vi "XVC_TX.vi"(6 "data in":string="shift:\u0005\u0000\u0000\u0000ÿ\u0000", 7 "Read (TRUE)":bool, 8 "error in":errorcluster, 9 "Address":u32=64 format="%.0x", 10 "IP address":string="192.168.10.20", 11 "connection ID":refnum<k16>) -> (0 "error out":errorcluster, 2 "received string":string, 3 "connection ID 2":refnum<k16>)   [LabVIEW 2017]
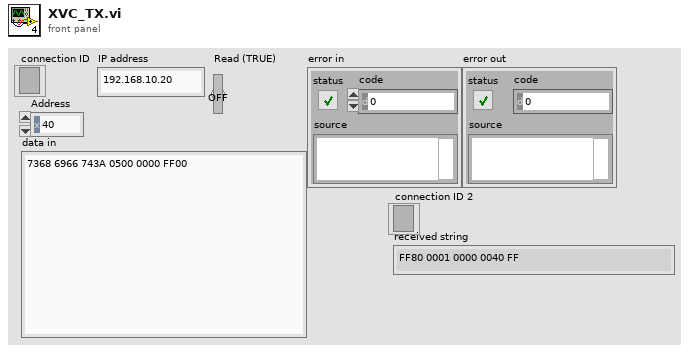
[diagram p1: front panel]
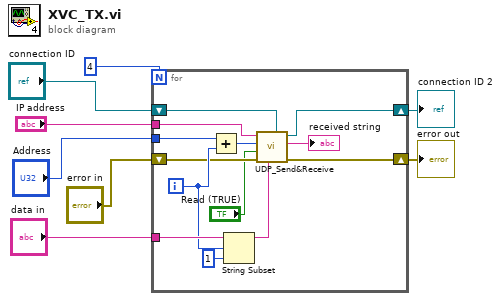
[diagram p0: block diagram]
diagram:
  n1 = for {
    N: 4 -> [_]
    shift-right: [w20] -> w2
    shift-left: "connection ID" -> [w21]
    tunnel: "Address" -> [w18]
    tunnel: "data in" -> [w17]
    shift-right: [w13] -> w3
    shift-left: "error in" -> [w12]
    tunnel: "IP address" -> [w11]
    i -> [w14]
    n2 = Add(x=w18, y=w14) -> (x+y=w19:u32)
    n3 = String Subset(string=w17, offset (0)=w14, length (rest)=1 ("length (rest)")) -> (substring=w16:string)
    n4 = call "UDP_Send&Receive.vi"("connection ID"=w21, "In"=w16, "error in (no error)"=w12, "Read (TRUE)"="Read (TRUE)", "Address"=w19, "IP address"=w11) -> ("error out"=w13:errorcluster, "received string"=→"received string":string, "connection ID out"=w20:refnum<k16>)  [unwired: 1 in, 1 out]
  }
  "error out" <- w3
  "connection ID 2" <- w2
